vi "Write T controller configuration.vi"(8 "error in (no error)":errorcluster, 10 "Configuration":T1={"Record Channels"=["A"], "Add raw signal"=FALSE, "New set point"=0.0}, 11 "Temperature Controller Driver in":refnum<class "Temperature Controller Driver.lvclass">) -> (0 "error out":errorcluster, 3 "Temperature Controller Driver out":refnum<class "Temperature Controller Driver.lvclass">)   [LabVIEW 2016, in "Temperature Controller Driver.lvclass"]
uses:
  Temperature Controller Driver.lvclass
  C:/github/NHMFL_Core/Libraries/Instruments/Instrument Driver/Instrument Driver.lvclass
  T controller configuration.ctl
  Instrument Driver/Write User configuration.vi
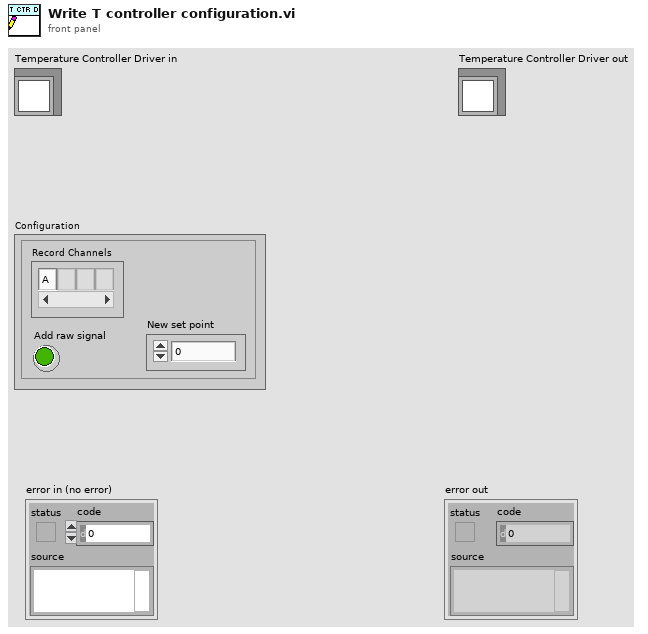
[diagram p1: front panel]
types:
  T1 = typedef "T controller configuration.ctl" = cluster{"Record Channels":string[], "Add raw signal":bool, "New set point":dbl}
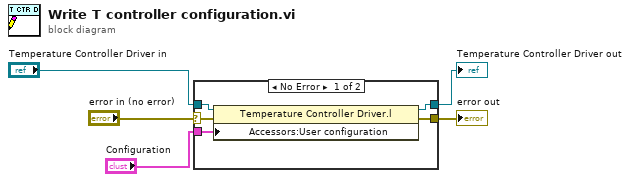
[diagram p0: block diagram]
diagram:
  n1 = case shown="No Error" "error in (no error)" {
    selector: "error in (no error)" -> [w8 w11]
    tunnel: [w7 w11] -> w4
    tunnel: [w6 w12] -> w2
    tunnel: "Temperature Controller Driver in" -> [w10 w12]
    tunnel: "Configuration" -> [w9 _]
    frame No Error {
      n2 = property class="Temperature Controller Driver.l"(reference=w10, error in=w8, "Accessors:User configuration"=w9) -> (reference out=w6:refnum<class "Temperature Controller Driver.lvclass">, error out=w7:errorcluster)
    }
    frame Error {
    }
  }
  "error out" <- w4
  "Temperature Controller Driver out" <- w2
